vi "GlobalDeviceNum2.vi"() -> ()   [LabVIEW 2020]
panel:
  in  "设备选择2":refnum<visa-resource-name>="USB0::0x0017::0x0001::NI-VISA-10001::RAW"
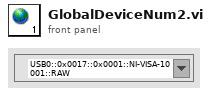
[diagram p1: front panel]
diagram:
